vi "Station 2.vi"(11 "IO":T1) -> (3 "bt_Node out":refnum<class "bt_Node.lvclass">)   [LabVIEW 2021, in "Car Wash Support.lvlib"]
uses:
  Car Wash Support.lvlib
  IO Refs.ctl
  <vilib>/TSA/Event Log/Event_TextLog/Event_TextLog.lvclass
  <vilib>/TSA/Abstract Data Classes/Abs_Types/Boolean/Abs_Boolean.lvclass
  C:/Program Files (x86)/National Instruments/LabVIEW 2021/vi.lib/TSA/Abstract Data Classes/Abs_Types/Value/Abs_Value.lvclass
  <vilib>/TSA/Abstract Data Classes/Abs_Types/I32 Integer/Abs_I32 Integer.lvclass
  <vilib>/TSA/Abstract Data Classes/Abs_Types/Double Float/Abs_Double Float.lvclass
  Wash Indicators.ctl
  Wash Options.ctl
  Support/Nodes/abs_Node/bt_Node.lvclass
  <vilib>/TSA/Abstract Data Classes/Constants/Support/Bool/Bool.vi
  BT.lvlib
  <vilib>/TSA/Abstract Data Classes/Constants/Support/Bool/Const_Bool.lvclass
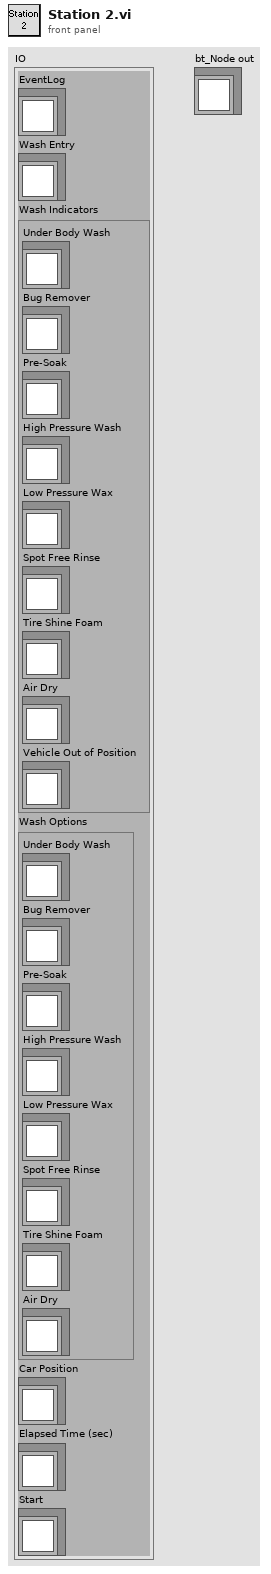
[diagram p1: front panel]
types:
  T1 = typedef "Car Wash Support.lvlib/IO Refs.ctl" = cluster{"EventLog":refnum<class "Event_TextLog.lvclass">, "Wash Entry":refnum<class "Abs_Boolean.lvclass">, "Wash Indicators":T2, "Wash Options":T3, "Car Position":refnum<class "Abs_I32 Integer.lvclass">, "Elapsed Time (sec)":refnum<class "Abs_Double Float.lvclass">, "Start":refnum<class "Abs_Boolean.lvclass">}
  T2 = typedef "Car Wash Support.lvlib/Wash Indicators.ctl" = cluster{"Under Body Wash":refnum<class "Abs_Boolean.lvclass">, "Bug Remover":refnum<class "Abs_Boolean.lvclass">, "Pre-Soak":refnum<class "Abs_Boolean.lvclass">, "High Pressure Wash":refnum<class "Abs_Boolean.lvclass">, "Low Pressure Wax":refnum<class "Abs_Boolean.lvclass">, "Spot Free Rinse":refnum<class "Abs_Boolean.lvclass">, "Tire Shine Foam":refnum<class "Abs_Boolean.lvclass">, "Air Dry":refnum<class "Abs_Boolean.lvclass">, "Vehicle Out of Position":refnum<class "Abs_Boolean.lvclass">}
  T3 = typedef "Car Wash Support.lvlib/Wash Options.ctl" = cluster{"Under Body Wash":refnum<class "Abs_Boolean.lvclass">, "Bug Remover":refnum<class "Abs_Boolean.lvclass">, "Pre-Soak":refnum<class "Abs_Boolean.lvclass">, "High Pressure Wash":refnum<class "Abs_Boolean.lvclass">, "Low Pressure Wax":refnum<class "Abs_Boolean.lvclass">, "Spot Free Rinse":refnum<class "Abs_Boolean.lvclass">, "Tire Shine Foam":refnum<class "Abs_Boolean.lvclass">, "Air Dry":refnum<class "Abs_Boolean.lvclass">}
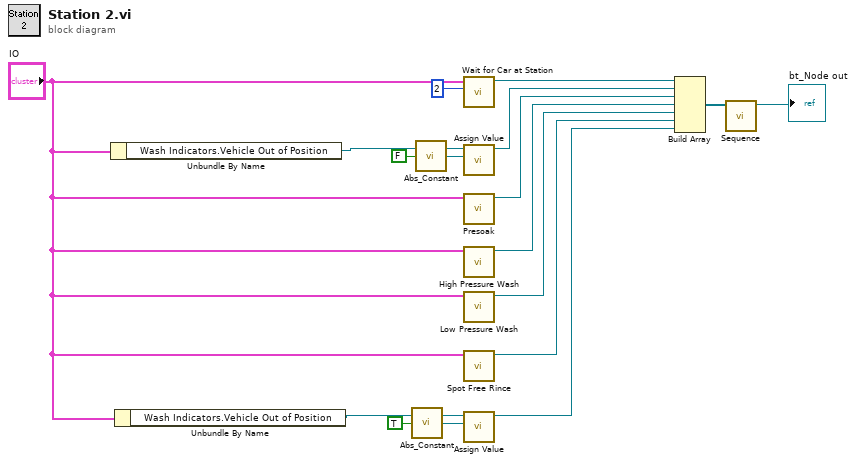
[diagram p0: block diagram]
diagram:
  n1 = Unbundle By Name("IO") -> ("Wash Indicators.Vehicle Out of Position"=w9:refnum<class "Abs_Boolean.lvclass">)
  n2 = Unbundle By Name("IO") -> ("Wash Indicators.Vehicle Out of Position"=w10:refnum<class "Abs_Boolean.lvclass">)
  n3 = call-poly <vilib>:"Abs_Constant.vi"("Boolean"=TRUE) -> ("Abs_Boolean.lvclass"=w13:refnum<class "Abs_Boolean.lvclass">)  [unwired: 4 in]
  n4 = call-poly <vilib>:"Abs_Constant.vi"("Boolean"=FALSE) -> ("Abs_Boolean.lvclass"=w7:refnum<class "Abs_Boolean.lvclass">)  [unwired: 4 in]
  n5 = call "Wait for Car at Station.vi"("Station Number"=2 ("Station"), "IO"="IO") -> ("bt_Node out"=w2:refnum<class "bt_Node.lvclass">)  [unwired: 9 in]
  n6 = call "Assign Value.vi"("Assigned Value"=w7, "Value"=w9) -> ("Node Out"=w6:refnum<class "bt_Node.lvclass">)  [unwired: 9 in]
  n7 = call "Presoak.vi"("IO"="IO") -> ("bt_Node out"=w15:refnum<class "bt_Node.lvclass">)  [unwired: 10 in]
  n8 = call "High Pressure Wash.vi"("IO"="IO") -> ("bt_Node out"=w14:refnum<class "bt_Node.lvclass">)  [unwired: 10 in]
  n9 = call "Low Pressure Wash.vi"("IO"="IO") -> ("bt_Node out"=w5:refnum<class "bt_Node.lvclass">)  [unwired: 10 in]
  n10 = call "Spot Free Rince.vi"("IO"="IO") -> ("bt_Node out"=w4:refnum<class "bt_Node.lvclass">)  [unwired: 10 in]
  n11 = call "Assign Value.vi"("Assigned Value"=w13, "Value"=w10) -> ("Node Out"=w11:refnum<class "bt_Node.lvclass">)  [unwired: 9 in]
  n12 = Build Array(w2, w6, w15, w14, w5, w4, w11) -> (w17:refnum<class "bt_Node.lvclass">[])
  n13 = call "Sequence.vi"("Nodes"=w17) -> ("Node"=→"bt_Node out":refnum<class "bt_Node.lvclass">)  [unwired: 10 in]
